vi "Calibration Verify Date.vi"(8 "error in (no error)":errorcluster, 10 "Date Override\n(yyyy,mm,dd)":string, 11 "VISA resource name":refnum<visa-resource-name>) -> (0 "error out":errorcluster, 3 "VISA resource name out":refnum<visa-resource-name>)   [LabVIEW 2020, in "Keithley 2450.lvlib"]
doc: "Sets the calibration verify date."
uses:
  Keithley 2450.lvlib
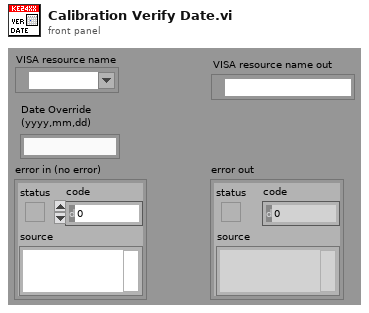
[diagram p1: front panel]
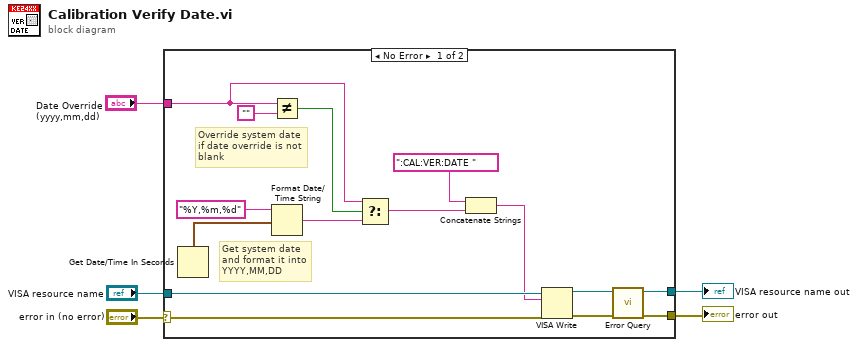
[diagram p0: block diagram]
diagram:
  n1 = case shown="No Error" "error in (no error)" {
    selector: "error in (no error)" -> [w20 w22]
    tunnel: [w9 w22] -> w4
    tunnel: "VISA resource name" -> [w19 w21]
    tunnel: [w8 w21] -> w2
    tunnel: "Date Override\n(yyyy,mm,dd)" -> [w10 _]
    frame No Error {
      # "Override system date if date override is not blank"
      # "Get system date and format it into\nYYYY,MM,DD"
      n2 = Get Date/Time In Seconds() -> (seconds since 1Jan1904=w14:timestamp)
      n3 = Not Equal?(x=w10, y="" ("x")) -> (x != y?=w15:bool)
      n4 = Format Date/Time String(time format string (%c)="%Y,%m,%d", seconds (now)=w14) -> (date/time string=w12:string)  [unwired: 1 out]
      n5 = Select(t=w10, s=w15, f=w12) -> (s? t:f=w13:string)
      n6 = Concatenate Strings(":CAL:VER:DATE " ("string"), w13) -> (w16:string)
      n7 = VISA Write(VISA resource name=w19, write buffer=w16, error in (no error)=w20) -> (VISA resource name out=w7:refnum<visa-resource-name>, error out=w6:errorcluster)  [unwired: 1 out]
      n8 = call "Error Query.vi"("error in (no error)"=w6, "VISA resource name"=w7) -> ("error out"=w9:errorcluster, "VISA resource name out"=w8:refnum<visa-resource-name>)  [unwired: 6 in, 2 out]
    }
    frame Error {
      # "Do nothing if error condition"
    }
  }
  "error out" <- w4
  "VISA resource name out" <- w2
